vi "Close.vi"(8 "error in":errorcluster, 11 "tcp server in":refnum<class "RT FlexRIO Server TCP.lvclass">) -> (0 "error out":errorcluster, 3 "tcp server out":refnum<class "RT FlexRIO Server TCP.lvclass">)   [LabVIEW 2017, in "RT FlexRIO Server TCP.lvclass"]
uses:
  RT FlexRIO Server TCP.lvclass
  RT FlexRIO Server TCP.lvclass/RT FlexRIO Server TCP.ctl
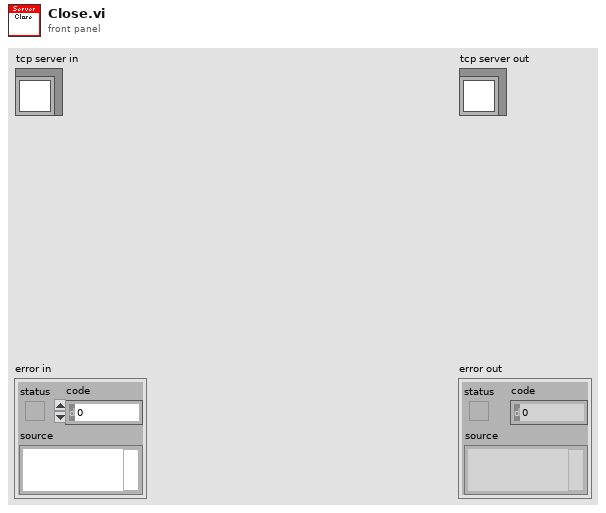
[diagram p1: front panel]
types:
  T1 = typedef "RT FlexRIO Server TCP.lvclass/SessionData.ctl" = cluster{"listener":refnum<k5>, "connection":refnum<k5>, "state":T2, "incoming":refnum<queue>, "outgoing":refnum<queue>, "state request":refnum<user-event>, "state changed":refnum<user-event>}
  T2 = typedef "RT FlexRIO Server TCP.lvclass/connection state.ctl" = enum16{"started", "connected", "stopped"}
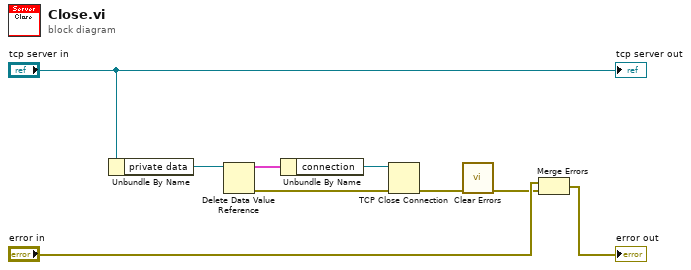
[diagram p0: block diagram]
diagram:
  n1 = Unbundle By Name("tcp server in") -> ("private data"=w8:refnum<data-value>)
  n2 = Delete Data Value Reference(data value reference=w8) -> (data value=w7:T1, error out=w4:errorcluster)  [unwired: 1 in]
  n3 = Unbundle By Name(w7) -> ("connection"=w6:refnum<k5>)
  n4 = TCP Close Connection(connection ID=w6, error in (no error)=w4) -> (error out=w3:errorcluster)  [unwired: 1 in, 1 out]
  n5 = call <vilib>:"Clear Errors.vi"("error in (no error)"=w3) -> ("error out"=w1:errorcluster)  [unwired: 5 in, 1 out]
  n6 = Merge Errors("error in", w1) -> (→"error out":errorcluster)
  "tcp server out" <- "tcp server in"
